vi "Run.vi"(8 "error in (no error)":errorcluster, 11 "socket REQ in":refnum<class "socket REQ.lvclass">) -> (0 "error out":errorcluster, 3 "socket REQ out":refnum<class "socket REQ.lvclass">)   [LabVIEW 2018, in "socket REQ.lvclass"]
uses:
  socket REQ.lvclass
  C:/Users/Denis/Desktop/S4ACS/S4ACS/communication-manager/Socket/Socket.lvclass
  Socket/Socket.lvclass
  State Machine/CM_State Machine.lvclass
  RxTx/CM_RxTx.lvclass
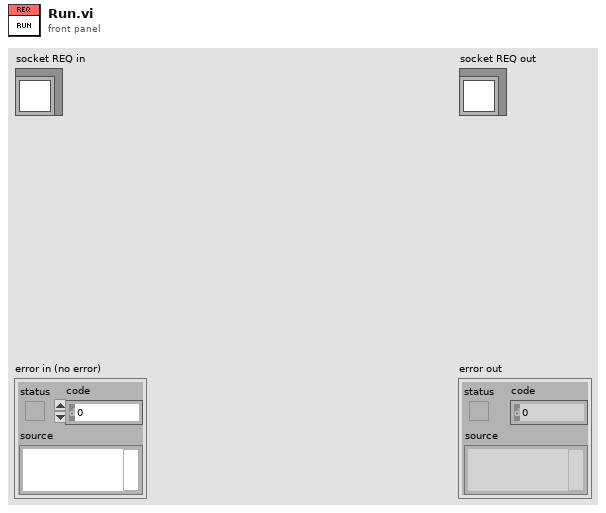
[diagram p1: front panel]
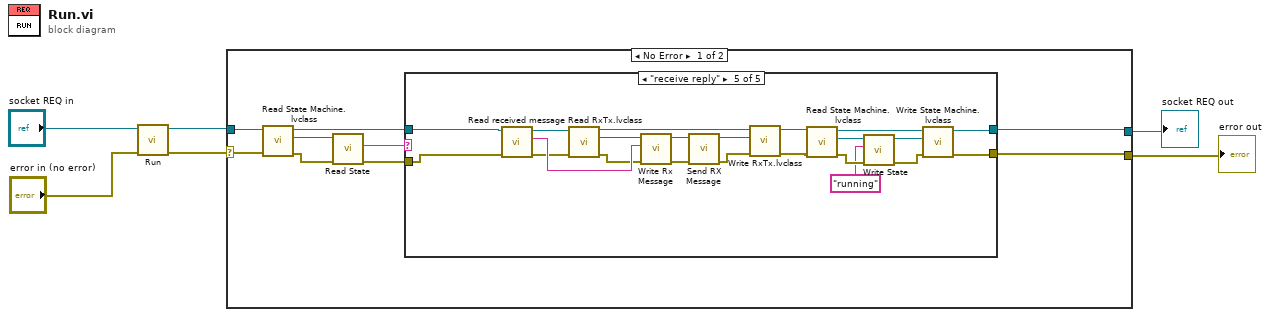
[diagram p0: block diagram]
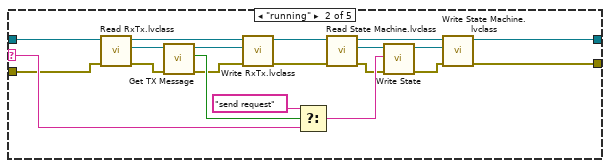
[diagram p3: hidden frame]
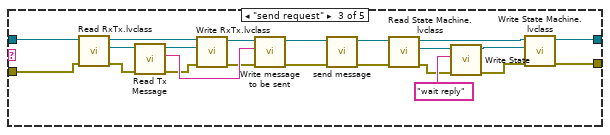
[diagram p4: hidden frame]
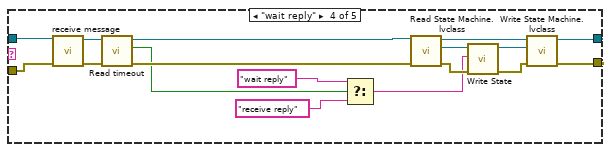
[diagram p5: hidden frame]
diagram:
  n1 = call-parent "Run.vi"("error in (no error)"="error in (no error)", "Socket in"="socket REQ in") -> ("error out"=w3:errorcluster, "Socket out"=w4:refnum<class "socket REQ.lvclass">)  [unwired: 8 in]
  n2 = case shown="No Error" w3 {
    selector: w3 -> [w11 w99]
    tunnel: w4 -> [w9 w100]
    tunnel: [w7 w100] -> w2
    tunnel: [w10 w99] -> w1
    frame No Error {
      n3 = call-dynamic "Read State Machine.lvclass.vi"("error in (no error)"=w11, "Socket in"=w9) -> ("error out"=w13:errorcluster, "CM_State Machine.lvclass"=w15:refnum<class "CM_State Machine.lvclass">, "Socket out"=w8:refnum<class "socket REQ.lvclass">)  [unwired: 7 in]
      n4 = call-dynamic "Read State.vi"("error in (no error)"=w13, "State Machine in"=w15) -> ("error out"=w12:errorcluster, "State"=w14:string)  [unwired: 7 in, 1 out]
      n5 = case shown="\"receive reply\"" w14 {
        selector: w14 -> [_ w36 _ _ _]
        tunnel: w8 -> [w17 w24 w56 w75 w78]
        tunnel: [w17 w18 w50 w69 w80] -> w7
        tunnel: [w16 w27 w49 w68 w79] -> w10
        tunnel: w12 -> [w16 w34 w55 w76 w77]
        frame Default {
        }
        frame "running" {
          n6 = call-dynamic "Read RxTx.lvclass.vi"("error in (no error)"=w34, "Socket in"=w24) -> ("error out"=w30:errorcluster, "CM_RxTx.lvclass"=w32:refnum<class "CM_RxTx.lvclass">, "Socket out"=w23:refnum<class "socket REQ.lvclass">)  [unwired: 7 in]
          n7 = call "Get TX Message.vi"("error in (no error)"=w30, "RxTx in"=w32) -> ("error out"=w29:errorcluster, "New msg"=w37:bool, "RxTx out"=w31:refnum<class "CM_RxTx.lvclass">)  [unwired: 7 in]
          n8 = call-dynamic "Write RxTx.lvclass.vi"("error in (no error)"=w29, "CM_RxTx.lvclass"=w31, "Socket in"=w23) -> ("error out"=w26:errorcluster, "Socket out"=w22:refnum<class "socket REQ.lvclass">)  [unwired: 7 in]
          n9 = Select(t="send request", s=w37, f=w36) -> (s? t:f=w33:string)
          n10 = call-dynamic "Read State Machine.lvclass.vi"("error in (no error)"=w26, "Socket in"=w22) -> ("error out"=w25:errorcluster, "CM_State Machine.lvclass"=w20:refnum<class "CM_State Machine.lvclass">, "Socket out"=w21:refnum<class "socket REQ.lvclass">)  [unwired: 7 in]
          n11 = call-dynamic "Write State.vi"("error in (no error)"=w25, "State"=w33, "State Machine in"=w20) -> ("error out"=w28:errorcluster, "State Machine out"=w19:refnum<class "CM_State Machine.lvclass">)  [unwired: 7 in]
          n12 = call-dynamic "Write State Machine.lvclass.vi"("error in (no error)"=w28, "CM_State Machine.lvclass"=w19, "Socket in"=w21) -> ("error out"=w27:errorcluster, "Socket out"=w18:refnum<class "socket REQ.lvclass">)  [unwired: 7 in]
        }
        frame "send request" {
          n13 = call-dynamic "Read RxTx.lvclass.vi"("error in (no error)"=w55, "Socket in"=w56) -> ("error out"=w40:errorcluster, "CM_RxTx.lvclass"=w54:refnum<class "CM_RxTx.lvclass">, "Socket out"=w45:refnum<class "socket REQ.lvclass">)  [unwired: 7 in]
          n14 = call "Read Tx Message.vi"("error in (no error)"=w40, "RxTx in"=w54) -> ("error out"=w42:errorcluster, "Tx Message"=w57:string, "RxTx out"=w41:refnum<class "CM_RxTx.lvclass">)  [unwired: 7 in]
          n15 = call-dynamic "Write RxTx.lvclass.vi"("error in (no error)"=w42, "CM_RxTx.lvclass"=w41, "Socket in"=w45) -> ("error out"=w43:errorcluster, "Socket out"=w44:refnum<class "socket REQ.lvclass">)  [unwired: 7 in]
          n16 = call-dynamic "Write message to be sent.vi"("error in (no error)"=w43, "message to be sent"=w57, "Socket in"=w44) -> ("error out"=w58:errorcluster, "Socket out"=w59:refnum<class "socket REQ.lvclass">)  [unwired: 7 in]
          n17 = call "send message.vi"("error in (no error)"=w58, "Socket in"=w59) -> ("error out"=w38:errorcluster, "Socket out"=w39:refnum<class "socket REQ.lvclass">)  [unwired: 8 in]
          n18 = call-dynamic "Read State Machine.lvclass.vi"("error in (no error)"=w38, "Socket in"=w39) -> ("error out"=w48:errorcluster, "CM_State Machine.lvclass"=w47:refnum<class "CM_State Machine.lvclass">, "Socket out"=w46:refnum<class "socket REQ.lvclass">)  [unwired: 7 in]
          n19 = call-dynamic "Write State.vi"("error in (no error)"=w48, "State"="wait reply" ("new state"), "State Machine in"=w47) -> ("error out"=w51:errorcluster, "State Machine out"=w52:refnum<class "CM_State Machine.lvclass">)  [unwired: 7 in]
          n20 = call-dynamic "Write State Machine.lvclass.vi"("error in (no error)"=w51, "CM_State Machine.lvclass"=w52, "Socket in"=w46) -> ("error out"=w49:errorcluster, "Socket out"=w50:refnum<class "socket REQ.lvclass">)  [unwired: 7 in]
        }
        frame "wait reply" {
          n21 = call-dynamic "receive message.vi"("error in (no error)"=w76, "Socket in"=w75) -> ("error out"=w66:errorcluster, "Socket out"=w67:refnum<class "socket REQ.lvclass">)  [unwired: 8 in]
          n22 = call-dynamic "Read timeout.vi"("error in (no error)"=w66, "Socket in"=w67) -> ("error out"=w64:errorcluster, "timeout"=w63:bool, "Socket out"=w65:refnum<class "socket REQ.lvclass">)  [unwired: 7 in]
          n23 = Select(t="wait reply" ("new state"), s=w63, f="receive reply" ("new state")) -> (s? t:f=w60:string)
          n24 = call-dynamic "Read State Machine.lvclass.vi"("error in (no error)"=w64, "Socket in"=w65) -> ("error out"=w72:errorcluster, "CM_State Machine.lvclass"=w71:refnum<class "CM_State Machine.lvclass">, "Socket out"=w70:refnum<class "socket REQ.lvclass">)  [unwired: 7 in]
          n25 = call-dynamic "Write State.vi"("error in (no error)"=w72, "State"=w60, "State Machine in"=w71) -> ("error out"=w73:errorcluster, "State Machine out"=w74:refnum<class "CM_State Machine.lvclass">)  [unwired: 7 in]
          n26 = call-dynamic "Write State Machine.lvclass.vi"("error in (no error)"=w73, "CM_State Machine.lvclass"=w74, "Socket in"=w70) -> ("error out"=w68:errorcluster, "Socket out"=w69:refnum<class "socket REQ.lvclass">)  [unwired: 7 in]
        }
        frame "receive reply" {
          n27 = call-dynamic "Read received message.vi"("error in (no error)"=w77, "Socket in"=w78) -> ("error out"=w90:errorcluster, "received message"=w98:string, "Socket out"=w91:refnum<class "socket REQ.lvclass">)  [unwired: 7 in]
          n28 = call-dynamic "Read RxTx.lvclass.vi"("error in (no error)"=w90, "Socket in"=w91) -> ("error out"=w89:errorcluster, "CM_RxTx.lvclass"=w95:refnum<class "CM_RxTx.lvclass">, "Socket out"=w94:refnum<class "socket REQ.lvclass">)  [unwired: 7 in]
          n29 = call "Write Rx Message.vi"("error in (no error)"=w89, "Rx Message"=w98, "RxTx in"=w95) -> ("error out"=w96:errorcluster, "RxTx out"=w97:refnum<class "CM_RxTx.lvclass">)  [unwired: 7 in]
          n30 = call "Send RX Message.vi"("error in (no error)"=w96, "RxTx in"=w97) -> ("error out"=w92:errorcluster, "RxTx out"=w93:refnum<class "CM_RxTx.lvclass">)  [unwired: 8 in]
          n31 = call-dynamic "Write RxTx.lvclass.vi"("error in (no error)"=w92, "CM_RxTx.lvclass"=w93, "Socket in"=w94) -> ("error out"=w82:errorcluster, "Socket out"=w83:refnum<class "socket REQ.lvclass">)  [unwired: 7 in]
          n32 = call-dynamic "Read State Machine.lvclass.vi"("error in (no error)"=w82, "Socket in"=w83) -> ("error out"=w86:errorcluster, "CM_State Machine.lvclass"=w85:refnum<class "CM_State Machine.lvclass">, "Socket out"=w84:refnum<class "socket REQ.lvclass">)  [unwired: 7 in]
          n33 = call-dynamic "Write State.vi"("error in (no error)"=w86, "State"="running" ("new state"), "State Machine in"=w85) -> ("error out"=w87:errorcluster, "State Machine out"=w88:refnum<class "CM_State Machine.lvclass">)  [unwired: 7 in]
          n34 = call-dynamic "Write State Machine.lvclass.vi"("error in (no error)"=w87, "CM_State Machine.lvclass"=w88, "Socket in"=w84) -> ("error out"=w79:errorcluster, "Socket out"=w80:refnum<class "socket REQ.lvclass">)  [unwired: 7 in]
        }
      }
    }
    frame Error {
    }
  }
  "error out" <- w1
  "socket REQ out" <- w2
